vi "editroi.vi"(8 "error in":errorcluster, 9 "Calibration":T2, 10 "data ROIs":T1, 11 "Sum Spectrum":cluster{"Ramp Pattern":dbl[], "Array":i32[]}[](graph)) -> (0 "error out":errorcluster, 3 "data ROIs out":T1)   [LabVIEW 2023]
uses:
  control/rois list cluster.ctl
  control/param_calibrazione.ctl
  queue/Front Panel Message Queue.lvlib
panel:
  in  "ylog":bool
  in  "autoscale":bool
  out "ROI Max":dbl
  out "ROI Min":dbl
  in  "Action":u16(ring) items=["Add", "Edit", "Delete"]
  out "ROIs Values Data":dbl[][](array[numeric])
  in  "set":bool
  in  "Name New Element":string
  out "ROIs Values":string[][](table)
  in  "ROIs List":i16(ring) items=["All"=0, "Ca - Escape Peak"=1, "S - Ka1"=2, "Cl - Ka1"=3, "Ar - Ka1"=4, "K - Ka1"=5, "Ca - Ka1"=6, "Ca - Kb1"=7, "Ti - Ka1"=8, "Mn - Ka1"=10, "Fe - Ka1"=11, "Fe - Kb1"=12, "Cu - Ka1"=13, "Zn - Ka1"=14]
  in  "Stop":bool
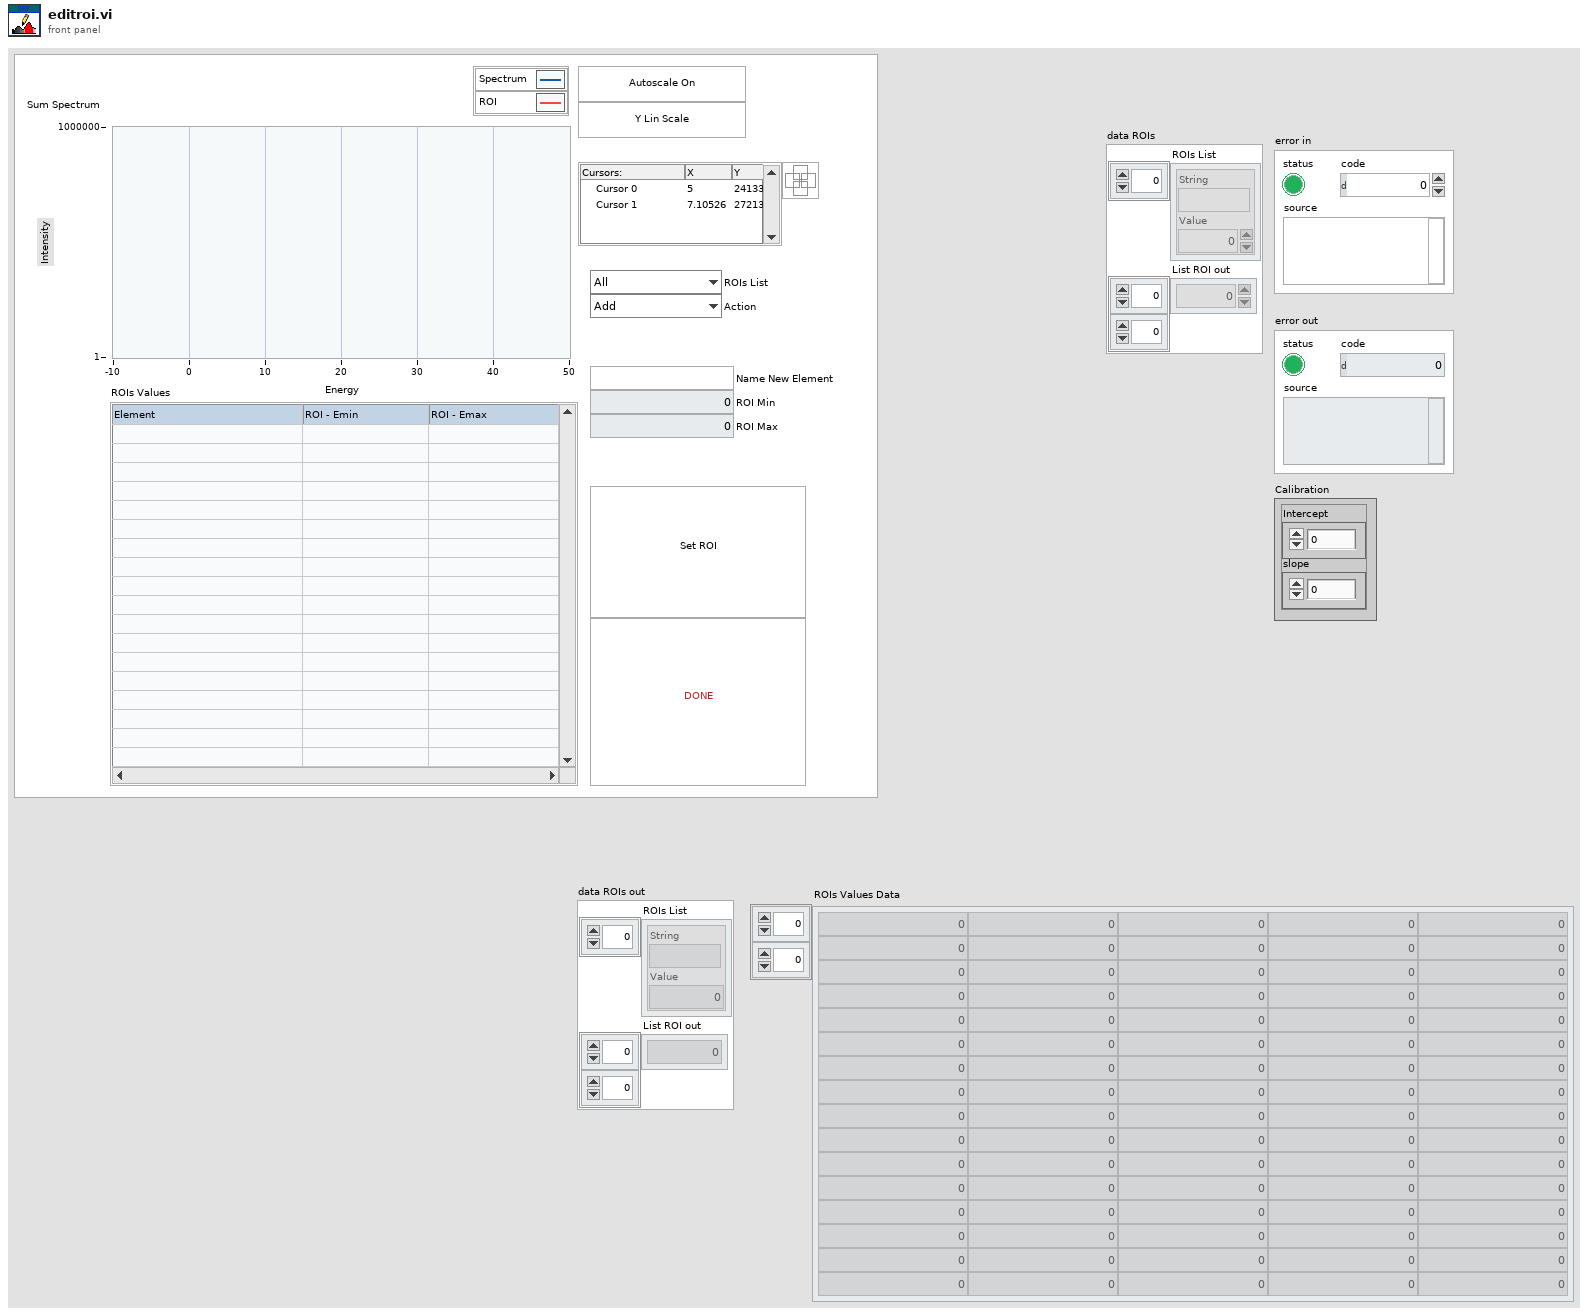
[diagram p1: front panel]
types:
  T1 = typedef "rois list cluster.ctl" = cluster{"ROIs List":cluster{"String":string, "Value":i32}[], "List ROI out":dbl[][]}
  T2 = typedef "param_calibrazione.ctl" = cluster{"Intercept":dbl, "slope":dbl}
  T3 = typedef "Front Panel Message Queue.lvlib/load Message Queues.ctl" = cluster{"Main":refnum<queue>}
  T4 = cluster{"Name New Element":string, "Cursor.Cursor X":dbl, "Cursor.Cursor X":dbl, "Action":u16, "ROI selected":i32}
  T5 = cluster{"Name New Element":string, "Cursor.Cursor X":dbl, "Cursor.Cursor X":dbl, "Action":u16, "ROIs List":i16}
  T6 = typedef "LVRowAndColumnTypeDef.ctl" = cluster{"Row":i32, "Column":i32}
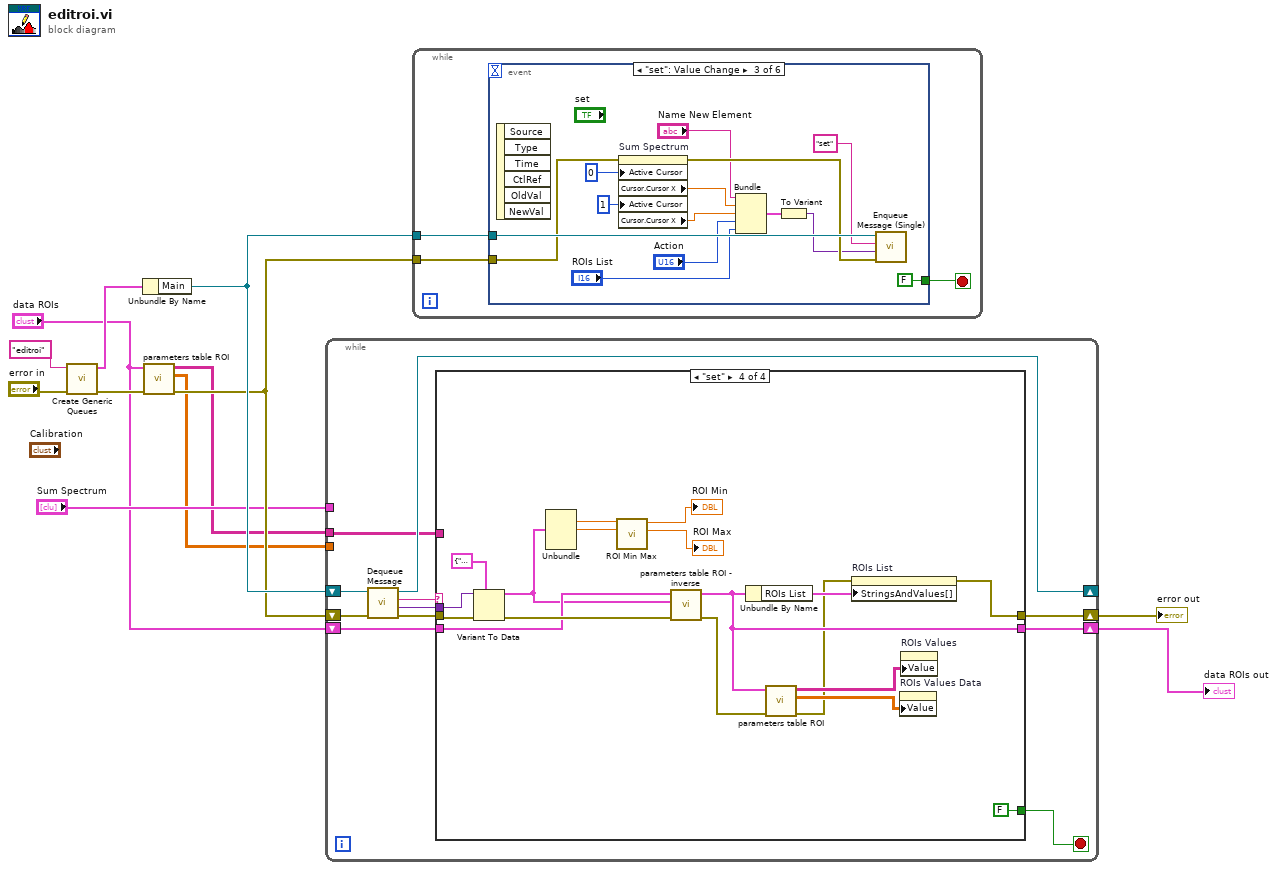
[diagram p0: block diagram]
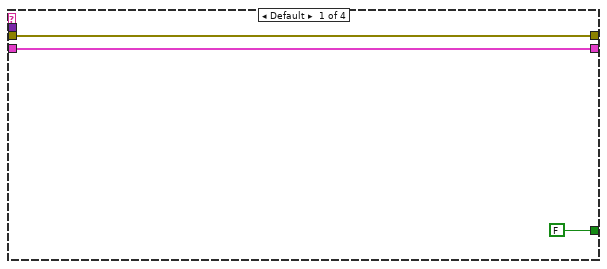
[diagram p2: hidden frame]
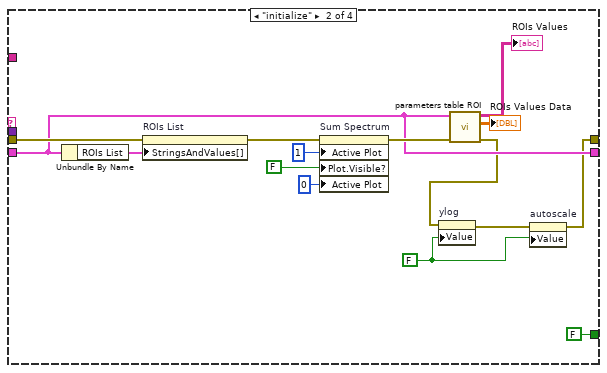
[diagram p3: hidden frame]
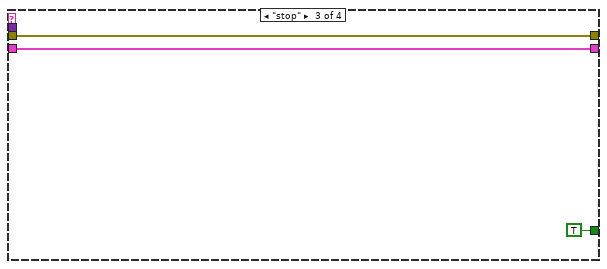
[diagram p4: hidden frame]
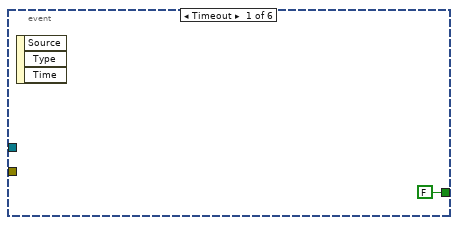
[diagram p5: hidden frame]
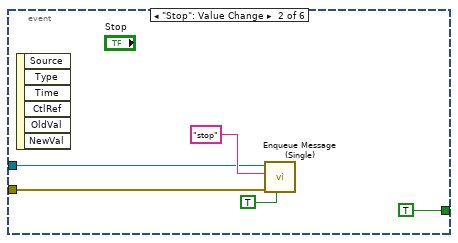
[diagram p6: hidden frame]
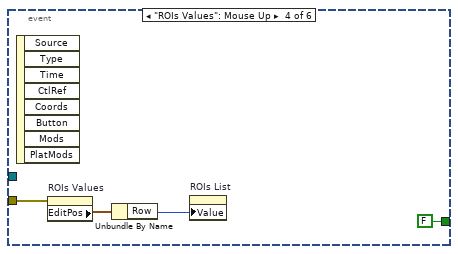
[diagram p7: hidden frame]
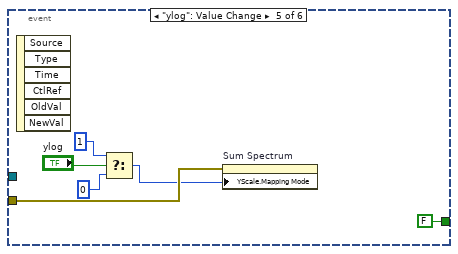
[diagram p8: hidden frame]
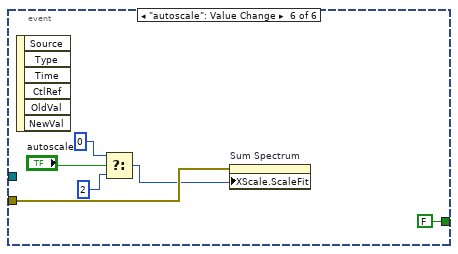
[diagram p9: hidden frame]
diagram:
  n1 = call "Create Generic Queues.vi"("error in (no error)"="error in", "name"="editroi") -> ("error out"=w10:errorcluster, "Message Queues"=w9:T3)  [unwired: 8 in]
  n2 = Unbundle By Name(w9) -> ("Main"=w8:refnum<queue>)
  n3 = call "parameters table ROI.vi"("error in"=w10, "data ROIs"="data ROIs") -> ("error out"=w7:errorcluster, "ROIs Values Data"=w3:dbl[][], "ROIs Values"=w4:string[][])  [unwired: 7 in]
  n4 = while {
    shift-right: [w17] -> _
    shift-left: w8 -> [w20]
    shift-right: [w18] -> w6
    shift-left: w7 -> [w21]
    tunnel: "Sum Spectrum" -> [_]
    tunnel: w4 -> [w13]
    tunnel: w3 -> [_]
    shift-right: [w14] -> w1
    shift-left: "data ROIs" -> [w16]
    stop <- w22 stop-if-true
    n5 = call "Dequeue Message.vi"("error in (no error)"=w21, "Message Queue"=w20) -> ("error out"=w19:errorcluster, "Message Data"=w15:variant, "Message"=w23:string, "dup Message Queue"=w17:refnum<queue>)  [unwired: 5 in, 1 out]
    n6 = case shown="\"set\"" w23 {
      tunnel: [FALSE FALSE TRUE FALSE] -> w22
      tunnel: w19 -> [w25 w41 w43 w61]
      tunnel: [w25 w28 w43 w56] -> w18
      tunnel: w16 -> [w24 w32 w42 w57]
      tunnel: w15 -> [_ _ _ w60]
      tunnel: [w24 w32 w42 w52] -> w14
      tunnel: w13 -> [_ _ _ _]
      frame Default {
      }
      frame "initialize" {
        w29 = FALSE ("ylog")
        n7 = Unbundle By Name(w32) -> ("ROIs List"=w39:cluster{"String":string, "Value":i32}[])
        n8 = property on="ROIs List" class="Ring (strict)"(error in=w41, "StringsAndValues[]"=w39) -> (error out=w38:errorcluster)  [unwired: 1 in, 1 out]
        n9 = property on="Sum Spectrum" class="XYGraph (strict)"(error in=w38, "Active Plot"=u32 1, "Plot.Visible?"=FALSE ("Plot.Visible"), "Active Plot"=u32 0) -> (error out=w34:errorcluster)  [unwired: 1 in, 1 out]
        n10 = call "parameters table ROI.vi"("error in"=w34, "data ROIs"=w32) -> ("error out"=w27:errorcluster, "ROIs Values Data"=→"ROIs Values Data":dbl[][], "ROIs Values"=→"ROIs Values":string[][])  [unwired: 7 in]
        n11 = property on="ylog" class="Bool (strict)"(error in=w27, "Value"=w29) -> (error out=w30:errorcluster)  [unwired: 1 in, 1 out]
        n12 = property on="autoscale" class="Bool (strict)"(error in=w30, "Value"=w29) -> (error out=w28:errorcluster)  [unwired: 1 in, 1 out]
      }
      frame "stop" {
      }
      frame "set" {
        n13 = Variant To Data(error in=w61, type=T4 {"Name New Element"="", "Cursor.Cursor X"=0.0, "Cursor.Cursor X"=0.0, "Action"=0, "ROI selected"=0} ("output cluster"), Variant=w60) -> (data=w49:T4, error out=w58:errorcluster)
        n14 = Unbundle(w49) -> ("Cursor.Cursor X"=w48:dbl, "Cursor.Cursor X"=w47:dbl)  [unwired: 3 out]
        n15 = call "ROI Min Max.vi"("ROI 2"=w47, "ROI 1"=w48) -> ("ROI Max"=→"ROI Max":dbl, "ROI Min"=→"ROI Min":dbl)  [unwired: 8 in]
        n16 = call "parameters table ROI - inverse.vi"("error in"=w58, "Edit Cluster"=w49, "data ROIs In"=w57) -> ("error out"=w51:errorcluster, "data ROIs Out"=w52:T1)  [unwired: 7 in]
        n17 = Unbundle By Name(w52) -> ("ROIs List"=w55:cluster{"String":string, "Value":i32}[])
        n18 = call "parameters table ROI.vi"("error in"=w51, "data ROIs"=w52) -> ("error out"=w50:errorcluster, "ROIs Values Data"=w54:dbl[][], "ROIs Values"=w53:string[][])  [unwired: 7 in]
        n19 = property on="ROIs List" class="Ring (strict)"(error in=w50, "StringsAndValues[]"=w55) -> (error out=w56:errorcluster)  [unwired: 1 in, 1 out]
        n20 = property on="ROIs Values Data" class="Arr (strict)"("Value"=w54) -> ()  [unwired: 2 in, 2 out]
        n21 = property on="ROIs Values" class="Tbl (strict)"("Value"=w53) -> ()  [unwired: 2 in, 2 out]
      }
    }
  }
  "error out" <- w6
  "data ROIs out" <- w1
  n22 = while {
    tunnel: w8 -> [w64]
    tunnel: w7 -> [w63]
    stop <- w65 stop-if-true
    n23 = event shown="[2] \"set\": Value Change" {
      selector: _ -> [_ _ _ _ _ _]
      dyn-events: _ -> [_ _ _ _ _ _]
      timeout: _ -> [_ _ _ _ _ _]
      tunnel: [FALSE TRUE FALSE FALSE FALSE FALSE] -> w65
      tunnel: w64 -> [_ w69 w84 _ _ _]
      tunnel: w63 -> [_ w68 w81 w88 w94 w100]
      event Timeout {
        n24 = event-data() -> ()  [unwired: 1 in, 3 out]
      }
      event "Stop": Value Change {
        n25 = event-data() -> ()  [unwired: 1 in, 6 out]
        n26 = call "Enqueue Message (Single).vi"("Priority Message? (F)"=TRUE, "error in (no error)"=w68, "Message"="stop", "Message Queue"=w69) -> ()  [unwired: 6 in, 2 out]
      }
      event "set": Value Change {
        n27 = event-data() -> ()  [unwired: 1 in, 6 out]
        n28 = property on="Sum Spectrum" class="XYGraph (strict)"(error in=w81, "Active Cursor"=u32 0, "Active Cursor"=u32 1) -> (error out=w80:errorcluster, "Cursor.Cursor X"=w77:dbl, "Cursor.Cursor X"=w76:dbl)  [unwired: 1 in, 1 out]
        n29 = Bundle("Name New Element"="Name New Element", "Cursor.Cursor X"=w77, "Cursor.Cursor X"=w76, "Action"="Action", "ROIs List"="ROIs List") -> (w75:T5)  [unwired: 1 in]
        n30 = To Variant(anything=w75) -> (Variant=w74:variant)
        n31 = call "Enqueue Message (Single).vi"("error in (no error)"=w80, "Message Data"=w74, "Message"="set", "Message Queue"=w84) -> ()  [unwired: 6 in, 2 out]
      }
      event "ROIs Values": Mouse Up {
        n32 = event-data() -> ()  [unwired: 1 in, 8 out]
        n33 = property on="ROIs Values" class="Tbl (strict)"(error in=w88) -> ("EditPos"=w87:T6)  [unwired: 1 in, 2 out]
        n34 = Unbundle By Name(w87) -> ("Row"=w86:i32)
        n35 = property on="ROIs List" class="Ring (strict)"("Value"=w86) -> ()  [unwired: 2 in, 2 out]
      }
      event "ylog": Value Change {
        n36 = event-data() -> ()  [unwired: 1 in, 6 out]
        n37 = Select(t=1, s="ylog", f=0) -> (s? t:f=w90:i32)
        n38 = property on="Sum Spectrum" class="XYGraph (strict)"(error in=w94, "YScale.Mapping Mode"=w90) -> ()  [unwired: 1 in, 2 out]
      }
      event "autoscale": Value Change {
        n39 = event-data() -> ()  [unwired: 1 in, 6 out]
        n40 = Select(t=0, s="autoscale", f=2) -> (s? t:f=w97:i32)
        n41 = property on="Sum Spectrum" class="XYGraph (strict)"(error in=w100, "XScale.ScaleFit"=w97) -> ()  [unwired: 1 in, 2 out]
      }
    }
  }
